vi "robotkolkontrol.vi"() -> ()   [LabVIEW 2016]
uses:
  <vilib>/LabVIEW Interface for Arduino/LabVIEW Interface for Arduino.lvlib
panel:
  in  "çalışma hızı":dbl
  in  "stop":bool
  in  "Number of Servos":u8=2
  in  "x açısı2":dbl
  in  "y açısı2":dbl
  in  "x açısı":dbl
  in  "y açısı":dbl
  in  "motor1":dbl(knob) scale=0.0..150.0
  out "Servo 0":dbl(knob) scale=0.0..180.0
  out "Servo 1":dbl(knob) scale=0.0..150.0
  in  "motor 2":dbl(knob) scale=0.0..150.0
  out "Servo 2":dbl(knob) scale=0.0..90.0
  in  "açma-kapama":dbl(knob) scale=0.0..120.0
  in  "otomatik(aç)-manuel(kapa)":bool
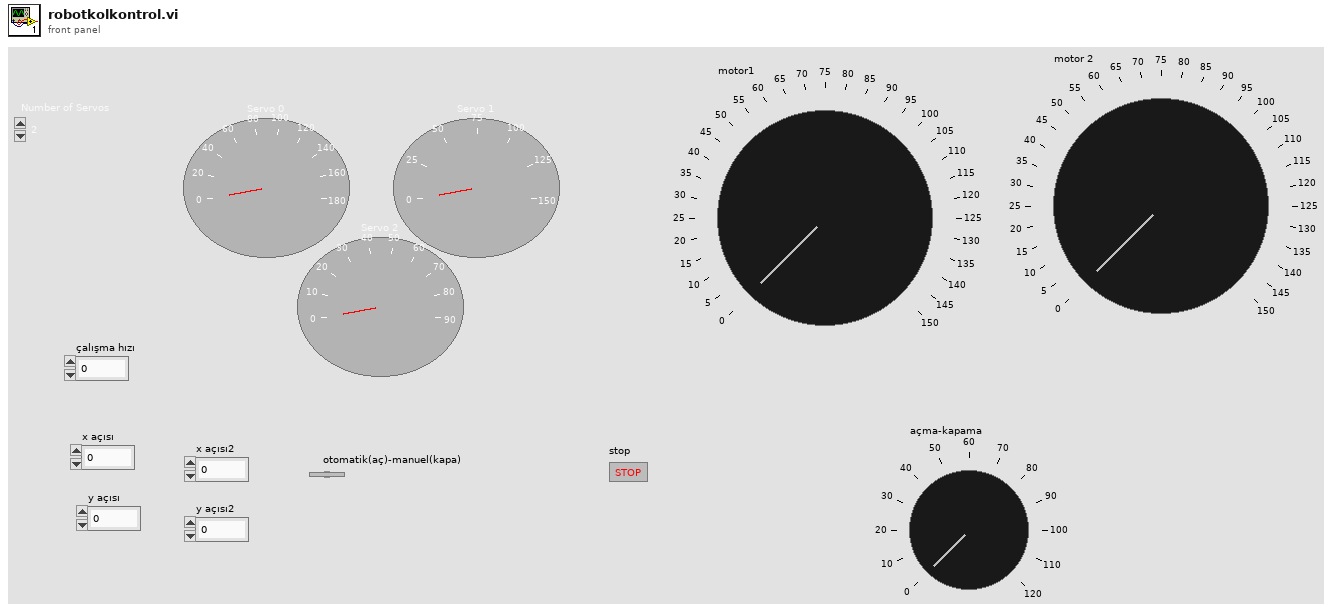
[diagram p1: front panel]
types:
  T1 = typedef "LabVIEW Interface for Arduino.lvlib/Arduino Resource.ctl" = cluster{"VISA resource":refnum<visa-resource-name>, "Board Type":T2, "Connection Type":enum8{"USB / Serial"}, "Bytes Per Packet (15)":u8}
  T2 = typedef "LabVIEW Interface for Arduino.lvlib/Board Type.ctl" = enum16{"Uno", "Dimuelanove w/Atmega 328", "Mega 2560"}
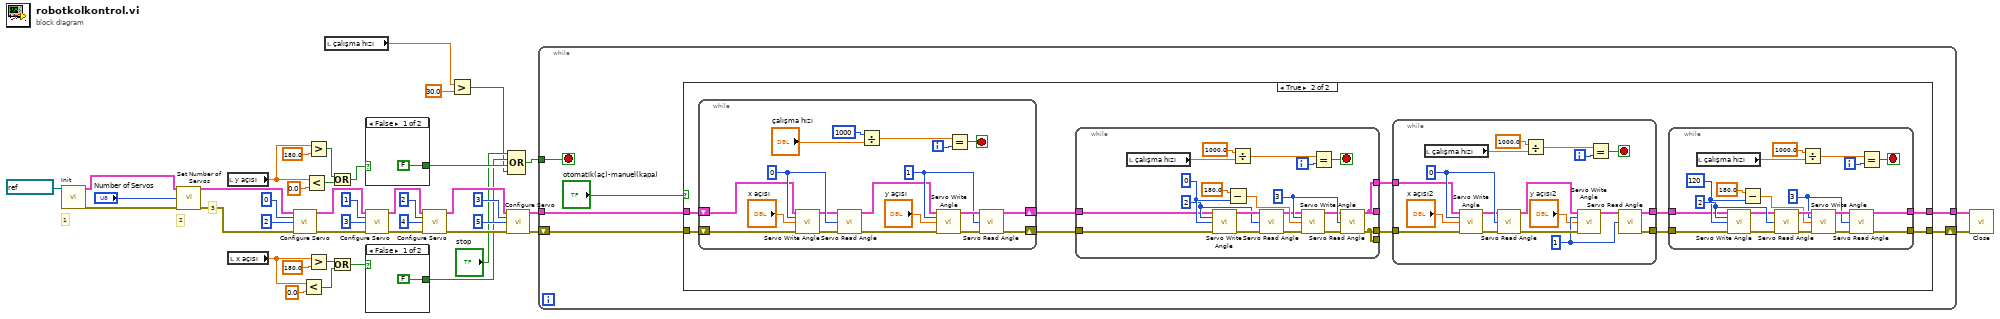
[diagram p0: block diagram]
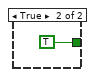
[diagram p2: hidden frame]
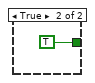
[diagram p3: hidden frame]
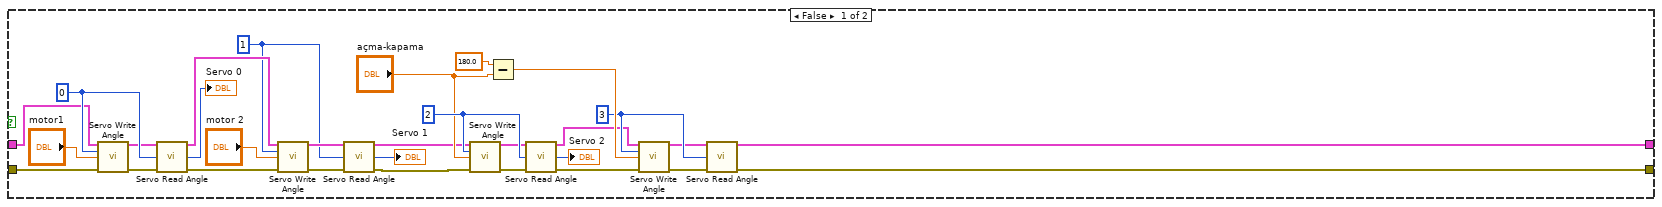
[diagram p4: hidden frame]
diagram:
  # "3"
  # "2"
  # "1"
  n1 = call <vilib>:"Init.vi"("VISA resource"=refnum<visa-resource-name> "COM3") -> ("Arduino Resource"=w43:T1, "error out"=w42:errorcluster)  [unwired: 17 in]
  n2 = call <vilib>:"Set Number of Servos.vi"("Arduino Resource"=w43, "Number Of Servos (1)"="Number of Servos", "error in"=w42) -> ("Arduino Resource"=w40:T1, "error out"=w39:errorcluster)  [unwired: 11 in]
  n3 = local read "y açısı"() -> (w11:dbl)
  n4 = local read "x açısı"() -> (w17:dbl)
  n5 = call <vilib>:"Configure Servo.vi"("Arduino Resource"=w40, "Servo Number (0)"=u8 0 ("Servo Number"), "DIO Pin (2)"=u8 2 ("Servo Number"), "error in"=w39) -> ("Arduino Resource"=w38:T1, "error out"=w37:errorcluster)  [unwired: 10 in]
  n6 = Less?(x=w17, y=0.0) -> (x < y?=w19:bool)
  n7 = Less?(x=w11, y=0.0) -> (x < y?=w13:bool)
  n8 = Greater?(x=w11, y=180.0) -> (0:w9:bool)
  n9 = Greater?(x=w17, y=180.0) -> (0:w16:bool)
  n10 = local read "çalışma hızı"() -> (w1:dbl)
  n11 = Or(x=w9, y=w13) -> (x .or. y?=w10:bool)
  n12 = Or(x=w16, y=w19) -> (x .or. y?=w15:bool)
  n13 = case shown="False" w10 {
    tunnel: [FALSE TRUE] -> w8
    frame False {
    }
    frame True {
    }
  }
  n14 = call <vilib>:"Configure Servo.vi"("Arduino Resource"=w38, "Servo Number (0)"=u8 1 ("Servo Number"), "DIO Pin (2)"=u8 3 ("Servo Number"), "error in"=w37) -> ("Arduino Resource"=w31:T1, "error out"=w30:errorcluster)  [unwired: 10 in]
  n15 = case shown="False" w15 {
    tunnel: [FALSE TRUE] -> w6
    frame False {
    }
    frame True {
    }
  }
  n16 = call <vilib>:"Configure Servo.vi"("Arduino Resource"=w31, "Servo Number (0)"=u8 2, "DIO Pin (2)"=u8 4, "error in"=w30) -> ("Arduino Resource"=w27:T1, "error out"=w26:errorcluster)  [unwired: 10 in]
  n17 = Greater?(x=w1, y=30.0) -> (0:w3:bool)
  n18 = call <vilib>:"Configure Servo.vi"("Arduino Resource"=w27, "Servo Number (0)"=u8 3, "DIO Pin (2)"=u8 5, "error in"=w26) -> ("Arduino Resource"=w25:T1, "error out"=w24:errorcluster)  [unwired: 10 in]
  n19 = Compound Arithmetic op=OR("stop", w6, w8, w3) -> (w4:bool)
  n20 = while {
    tunnel: w25 -> [w52]
    shift-right: [w49] -> w21
    shift-left: w24 -> [w51]
    tunnel: [w50] -> w20
    tunnel: w4 -> [w48]
    stop <- w48 stop-if-true
    n21 = case shown="True" "otomatik(aç)-manuel(kapa)" {
      tunnel: w52 -> [w79 w93]
      tunnel: w51 -> [w78 w92]
      tunnel: [w57 w91] -> w50
      tunnel: [w58 w90] -> w49
      frame False {
        w68 = u8 3 ("Servo Number")
        w63 = u8 2 ("Servo Number")
        w56 = u8 1 ("Servo Number")
        w83 = u8 0 ("Servo Number")
        n22 = call <vilib>:"Servo Write Angle.vi"("Arduino Resource"=w79, "Servo Number"=w83, "Angle (Degrees)"="motor1", "error in"=w78) -> ("Arduino Resource"=w81:T1, "error out"=w82:errorcluster)  [unwired: 10 in]
        n23 = call <vilib>:"Servo Read Angle.vi"("Arduino Resource"=w81, "Servo Number"=w83, "error in"=w82) -> ("Arduino Resource"=w73:T1, "Angle (Degrees)"=→"Servo 0":u8, "error out"=w72:errorcluster)  [unwired: 10 in]
        n24 = call <vilib>:"Servo Write Angle.vi"("Arduino Resource"=w73, "Servo Number"=w56, "Angle (Degrees)"="motor 2", "error in"=w72) -> ("Arduino Resource"=w76:T1, "error out"=w75:errorcluster)  [unwired: 10 in]
        n25 = call <vilib>:"Servo Read Angle.vi"("Arduino Resource"=w76, "Servo Number"=w56, "error in"=w75) -> ("Arduino Resource"=w55:T1, "Angle (Degrees)"=→"Servo 1":u8, "error out"=w54:errorcluster)  [unwired: 10 in]
        n26 = call <vilib>:"Servo Write Angle.vi"("Arduino Resource"=w55, "Servo Number"=w63, "Angle (Degrees)"="açma-kapama", "error in"=w54) -> ("Arduino Resource"=w61:T1, "error out"=w62:errorcluster)  [unwired: 10 in]
        n27 = Subtract(x=180.0, y="açma-kapama") -> (x-y=w69:dbl)
        n28 = call <vilib>:"Servo Read Angle.vi"("Arduino Resource"=w61, "Servo Number"=w63, "error in"=w62) -> ("Arduino Resource"=w64:T1, "Angle (Degrees)"=→"Servo 2":u8, "error out"=w65:errorcluster)  [unwired: 10 in]
        n29 = call <vilib>:"Servo Write Angle.vi"("Arduino Resource"=w64, "Servo Number"=w68, "Angle (Degrees)"=w69, "error in"=w65) -> ("Arduino Resource"=w66:T1, "error out"=w67:errorcluster)  [unwired: 10 in]
        n30 = call <vilib>:"Servo Read Angle.vi"("Arduino Resource"=w66, "Servo Number"=w68, "error in"=w67) -> ("Arduino Resource"=w57:T1, "error out"=w58:errorcluster)  [unwired: 10 in, 1 out]
      }
      frame True {
        n31 = while {
          shift-right: [w145] -> w87
          shift-left: w93 -> [w141]
          shift-right: [w144] -> w86
          shift-left: w92 -> [w140]
          i -> [w138]
          stop <- w146 stop-if-true
          w147 = u8 1 ("Servo Number")
          w152 = u8 0 ("Servo Number")
          n32 = call <vilib>:"Servo Write Angle.vi"("Arduino Resource"=w141, "Servo Number"=w152, "Angle (Degrees)"="x açısı", "error in"=w140) -> ("Arduino Resource"=w150:T1, "error out"=w151:errorcluster)  [unwired: 10 in]
          n33 = call <vilib>:"Servo Read Angle.vi"("Arduino Resource"=w150, "Servo Number"=w152, "error in"=w151) -> ("Arduino Resource"=w143:T1, "error out"=w142:errorcluster)  [unwired: 10 in, 1 out]
          n34 = Divide(x=1000, y="çalışma hızı") -> (x/y=w134:dbl)
          n35 = call <vilib>:"Servo Write Angle.vi"("Arduino Resource"=w143, "Servo Number"=w147, "Angle (Degrees)"="y açısı", "error in"=w142) -> ("Arduino Resource"=w149:T1, "error out"=w148:errorcluster)  [unwired: 10 in]
          n36 = Equal?(x=w134, y=w138) -> (x = y?=w146:bool)
          n37 = call <vilib>:"Servo Read Angle.vi"("Arduino Resource"=w149, "Servo Number"=w147, "error in"=w148) -> ("Arduino Resource"=w145:T1, "error out"=w144:errorcluster)  [unwired: 10 in, 1 out]
        }
        n38 = while {
          tunnel: [w98] -> _
          tunnel: [w97] -> _
          tunnel: w87 -> [w100]
          tunnel: w86 -> [w99]
          tunnel: [w98] -> w85
          tunnel: [w97] -> w84
          i -> [w102]
          stop <- w101 stop-if-true
          w105 = 0
          w104 = u8 2 ("Servo Number")
          w109 = u8 3 ("Servo Number")
          n39 = local read "çalışma hızı"() -> (w96:dbl)
          n40 = call <vilib>:"Servo Write Angle.vi"("Arduino Resource"=w100, "Servo Number"=w104, "Angle (Degrees)"=w105, "error in"=w99) -> ("Arduino Resource"=w108:T1, "error out"=w110:errorcluster)  [unwired: 10 in]
          n41 = Subtract(x=180.0, y=w105) -> (x-y=w113:dbl)
          n42 = Divide(x=1000.0, y=w96) -> (x/y=w95:dbl)
          n43 = call <vilib>:"Servo Read Angle.vi"("Arduino Resource"=w108, "Servo Number"=w104, "error in"=w110) -> ("Arduino Resource"=w107:T1, "error out"=w111:errorcluster)  [unwired: 10 in, 1 out]
          n44 = call <vilib>:"Servo Write Angle.vi"("Arduino Resource"=w107, "Servo Number"=w109, "Angle (Degrees)"=w113, "error in"=w111) -> ("Arduino Resource"=w106:T1, "error out"=w112:errorcluster)  [unwired: 10 in]
          n45 = Equal?(x=w95, y=w102) -> (x = y?=w101:bool)
          n46 = call <vilib>:"Servo Read Angle.vi"("Arduino Resource"=w106, "Servo Number"=w109, "error in"=w112) -> ("Arduino Resource"=w98:T1, "error out"=w97:errorcluster)  [unwired: 10 in, 1 out]
        }
        n47 = while {
          tunnel: [w159] -> w89
          tunnel: [w158] -> w88
          tunnel: w85 -> [w157]
          tunnel: w84 -> [w156]
          i -> [w166]
          stop <- w167 stop-if-true
          w161 = u8 1 ("Servo Number")
          w170 = u8 0 ("Servo Number")
          n48 = local read "çalışma hızı"() -> (w155:dbl)
          n49 = call <vilib>:"Servo Write Angle.vi"("Arduino Resource"=w157, "Servo Number"=w170, "Angle (Degrees)"="x açısı2", "error in"=w156) -> ("Arduino Resource"=w168:T1, "error out"=w169:errorcluster)  [unwired: 10 in]
          n50 = call <vilib>:"Servo Read Angle.vi"("Arduino Resource"=w168, "Servo Number"=w170, "error in"=w169) -> ("Arduino Resource"=w163:T1, "error out"=w162:errorcluster)  [unwired: 10 in, 1 out]
          n51 = Divide(x=1000.0, y=w155) -> (x/y=w153:dbl)
          n52 = call <vilib>:"Servo Write Angle.vi"("Arduino Resource"=w163, "Servo Number"=w161, "Angle (Degrees)"="y açısı2", "error in"=w162) -> ("Arduino Resource"=w164:T1)  [unwired: 10 in, 1 out]
          n53 = Equal?(x=w153, y=w166) -> (x = y?=w167:bool)
          n54 = call <vilib>:"Servo Read Angle.vi"("Arduino Resource"=w164, "Servo Number"=w161) -> ("Arduino Resource"=w159:T1, "error out"=w158:errorcluster)  [unwired: 11 in, 1 out]
        }
        n55 = while {
          tunnel: [w121] -> w91
          tunnel: [w120] -> w90
          tunnel: w89 -> [w118]
          tunnel: w88 -> [w117]
          i -> [w122]
          stop <- w123 stop-if-true
          w119 = 120
          w128 = u8 3 ("Servo Number")
          w130 = u8 2 ("Servo Number")
          n56 = local read "çalışma hızı"() -> (w116:dbl)
          n57 = call <vilib>:"Servo Write Angle.vi"("Arduino Resource"=w118, "Servo Number"=w130, "Angle (Degrees)"=w119, "error in"=w117) -> ("Arduino Resource"=w129:T1, "error out"=w127:errorcluster)  [unwired: 10 in]
          n58 = Subtract(x=180.0, y=w119) -> (x-y=w124:dbl)
          n59 = call <vilib>:"Servo Read Angle.vi"("Arduino Resource"=w129, "Servo Number"=w130, "error in"=w127) -> ("Arduino Resource"=w131:T1, "error out"=w126:errorcluster)  [unwired: 10 in, 1 out]
          n60 = Divide(x=1000.0, y=w116) -> (x/y=w114:dbl)
          n61 = call <vilib>:"Servo Write Angle.vi"("Arduino Resource"=w131, "Servo Number"=w128, "Angle (Degrees)"=w124, "error in"=w126) -> ("Arduino Resource"=w132:T1, "error out"=w125:errorcluster)  [unwired: 10 in]
          n62 = call <vilib>:"Servo Read Angle.vi"("Arduino Resource"=w132, "Servo Number"=w128, "error in"=w125) -> ("Arduino Resource"=w121:T1, "error out"=w120:errorcluster)  [unwired: 10 in, 1 out]
          n63 = Equal?(x=w114, y=w122) -> (x = y?=w123:bool)
        }
      }
    }
  }
  n64 = call <vilib>:"Close.vi"("Arduino Resource"=w20, "error in"=w21) -> ()  [unwired: 13 in, 1 out]
